vi "time + theta.vi"(5 "Draw Area Size":cluster{"Width":u32, "Height":u32}={"Width"=800, "Height"=90}, 6 "Sample volumes":dbl[unit][](array[numeric]) format="%.2f", 7 "colors":u32[](array[colorbox])=[16717824, 16775680, 65289, 1442031, 16711898, 9306367, 16711704, 16773418, 4914944, 65469, 18175, 15805183, 16711776, 16745216, 16773632, 7396352, 62719, 16383, 15925503, 16711686, 16775954, 65372, 51354, 19711, 7082751, 15663288, 16711680, 11468586, 52719, 1214975, 16711830], 8 "Sample start times":dbl[unit][](array[numeric]) format="%<%H:%M:%S>t", 9 "State Settings":T2[][](array[typedef]) {"valve cycle time" min=0.2 step=0.1 format="%.2f"; "flow division"."5" min=0.0 max=1.0 step=0.01 format="%.3f"; "flow division"."4" min=0.0 max=1.0 step=0.01 format="%.3f"; "flow division"."3" min=0.0 max=1.0 step=0.01 format="%.3f"; "flow division"."2" min=0.0 max=1.0 step=0.01 format="%.3f"; "flow division"."1" min=0.0 max=1.0 step=0.01 format="%.3f"; "flow rate" format="%.3f"}, 10 "Cycle list":i32(listbox), 11 "Method settings":T5 {"Column"."porosity" format="%.4f"; "Column"."diameter" format="%.2f"; "Column"."length" format="%.2f"}) -> (0 "Samples":T1, 2 "Sample plot":picture, 3 "tout":dbl[unit][](array[numeric]))   [LabVIEW 2012]
uses:
  Method settings.ctl
  Peristaltic/3-stop colors.ctl
  State Setting.ctl
  Stamp/Switch settings vertical.ctl
  flow fraction.ctl
  Samples.ctl
panel:
  out "f":dbl[](array[numeric])
  out "tcum":dbl[unit][](array[numeric])
  out "theta":dbl[unit][](array[numeric])
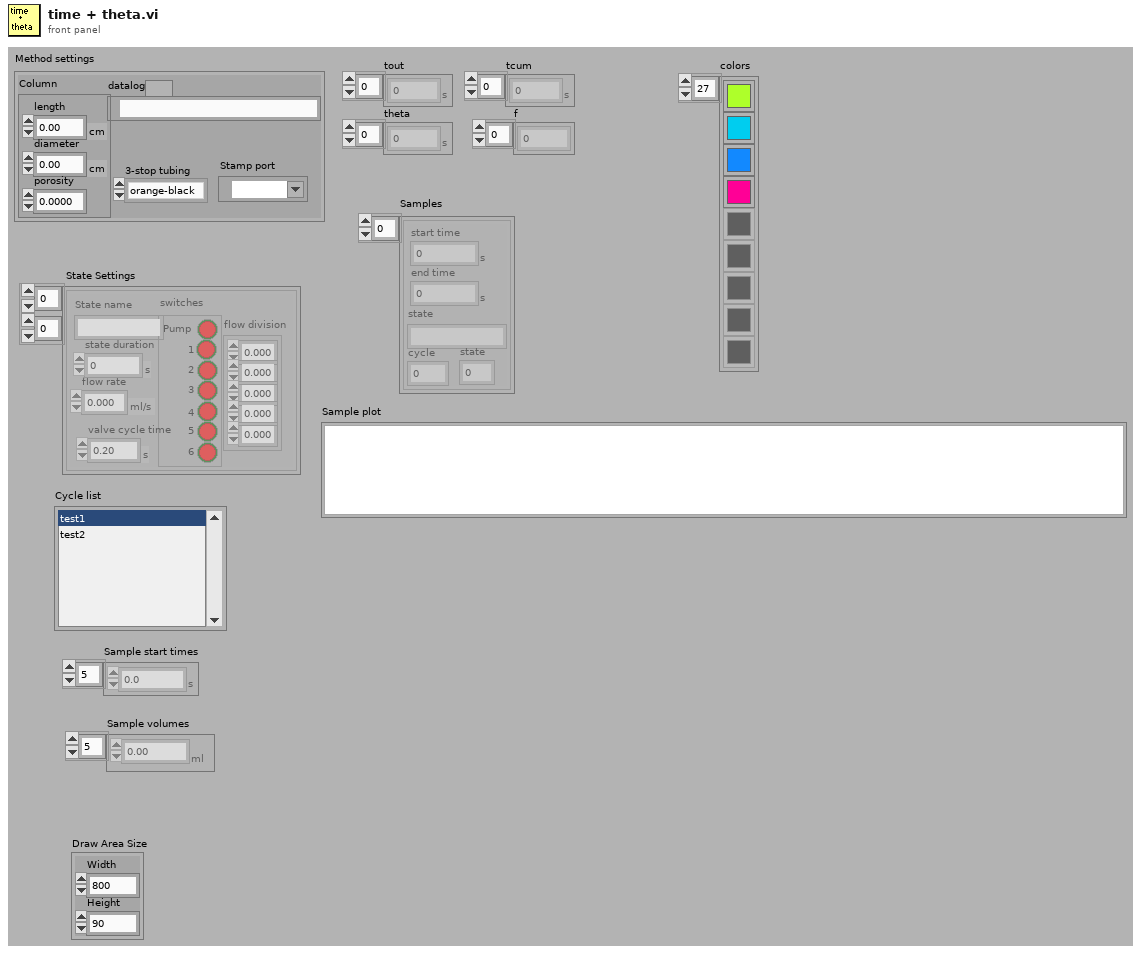
[diagram p1: front panel]
types:
  T1 = typedef "Samples.ctl" = cluster{"start time":dbl[unit], "end time":dbl[unit], "state":string, "cycle":u16, "state":u16}[]
  T2 = typedef "State Setting.ctl" = cluster{"switches":T3, "flow rate":dbl[unit], "flow division":cluster{"1":T4, "2":T4, "3":T4, "4":T4, "5":T4}, "State name":string, "state duration":dbl[unit], "valve cycle time":dbl[unit]}
  T3 = typedef "Switch settings vertical.ctl" = cluster{"Pump":bool, "1":bool, "2":bool, "3":bool, "4":bool, "5":bool, "6":bool}
  T4 = typedef "flow fraction.ctl" = dbl
  T5 = typedef "Method settings.ctl" = cluster{"3-stop tubing":T6, "Stamp port":refnum<visa-resource-name>, "datalog":path, "Column":cluster{"length":dbl[unit], "diameter":dbl[unit], "porosity":dbl}}
  T6 = typedef "3-stop colors.ctl" = enum16{"orange-black", "orange-red", "orange-blue", "orange-green", "green-yellow", "orange-yellow", "white-yellow", "orange-white", "black-black", "orange-orange", "white-black", "white-white", "white-red", "red-red", "red-grey", "grey-grey", "yellow-yellow", "yellow-blue", "blue-blue", "blue-green", "green-green", "purple-purple", "purple-black", "purple-orange", "purple-white", "black-white", "13", "14", "15", "16", "17", "18"}
  T7 = cluster{"Numeric":dbl[unit], dbl[unit], "State name":string, dbl, dbl}
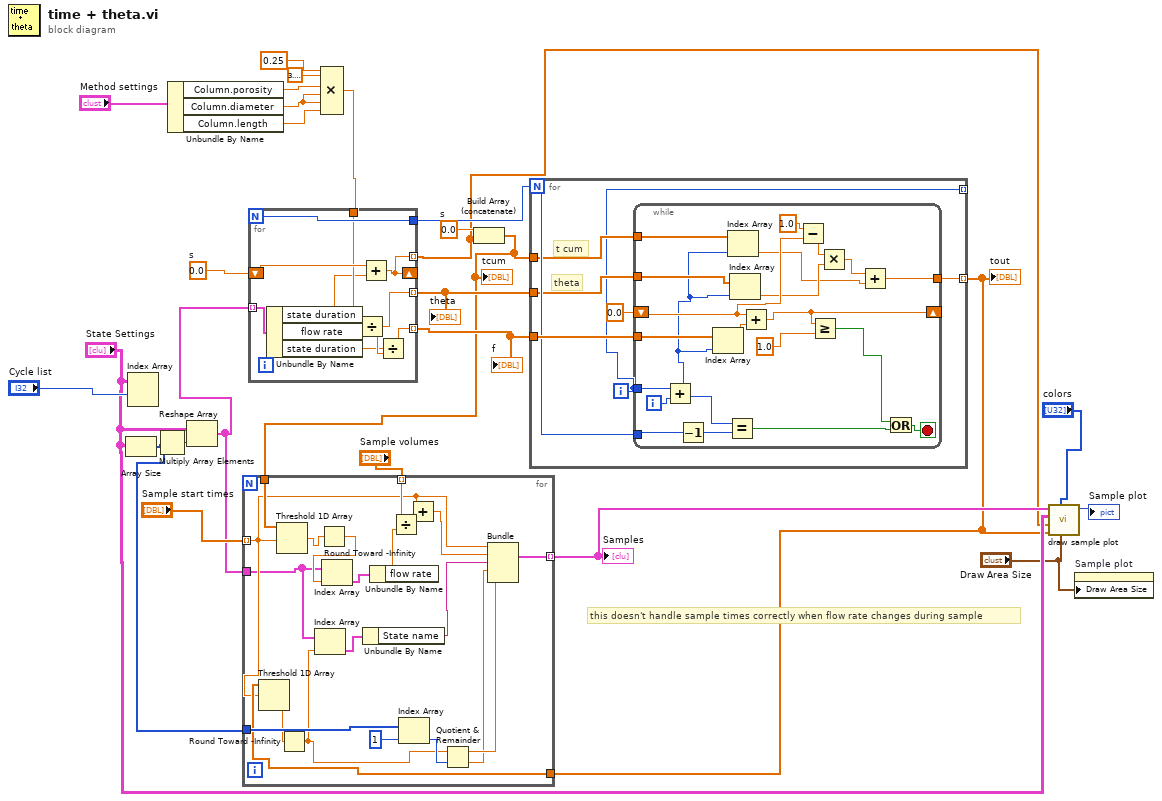
[diagram p0: block diagram]
diagram:
  w15 = dbl[unit] 0.0  # s
  w17 = dbl[unit] 0.0  # s
  # "this doesn't handle sample times correctly when flow rate changes during sample"
  n1 = Array Size(array="State Settings") -> (size(s)=w9:i32[])
  n2 = Index Array(array="State Settings", index (row)="Cycle list") -> ()  [unwired: 1 in, 1 out]
  n3 = Multiply Array Elements(1:w9) -> (0:w11:i32)
  n4 = Unbundle By Name("Method settings") -> ("Column.porosity"=w23:dbl, "Column.diameter"=w24:dbl[unit], "Column.length"=w25:dbl[unit])
  n5 = Reshape Array("State Settings", w11) -> (w10:T2[])
  n6 = Compound Arithmetic op=MULTIPLY(0.25 ("value"), 3.141592653589793, w23, w24, w24, w25) -> (w19:dbl[unit])
  n7 = for {
    N -> [w35]
    tunnel: w10 -> [w36] mode=indexing
    tunnel: w19 -> [w33]
    tunnel: [w32] -> w14 mode=indexing
    tunnel: [w35] -> w18
    shift-right: [w27] -> _
    shift-left: w17 -> [w34]
    tunnel: [w27] -> w4 mode=indexing
    tunnel: [w30] -> w16 mode=indexing
    n8 = Unbundle By Name(w36) -> ("state duration"=w31:dbl[unit], "flow rate"=w28:dbl[unit], "state duration"=w29:dbl[unit])
    n9 = Divide(x=w33, y=w28) -> (x/y=w30:dbl[unit])
    n10 = Add(x=w34, y=w31) -> (x+y=w27:dbl[unit])
    n11 = Divide(x=w29, y=w30) -> (x/y=w32:dbl)
  }
  "theta" <- w16
  "f" <- w14
  n12 = Build Array (concatenate)(w15, w4) -> (w3:dbl[unit][])
  "tcum" <- w3
  n13 = for {
    N: w18 -> [w42]
    tunnel: w14 -> [w43]
    tunnel: w3 -> [w40]
    tunnel: w16 -> [w39]
    tunnel: [w38] -> w2 mode=indexing
    tunnel: [w37] -> _ mode=indexing
    i -> [w37]
    # "t cum"
    # "theta"
    n14 = while {
      tunnel: w43 -> [w64]
      tunnel: w37 -> [w62]
      tunnel: w42 -> [w60]
      shift-right: [w46] -> _
      shift-left: 0.0 -> [w52]
      tunnel: w40 -> [w57]
      tunnel: w39 -> [w56]
      tunnel: [w55] -> w38
      i -> [w63]
      stop <- w61 stop-if-true
      n15 = Add(x=w62, y=w63) -> (x+y=w51:i32)
      n16 = Decrement(x=w60) -> (x-1=w54:i32)
      n17 = Index Array(array=w64, index=w51) -> (element=w58:dbl)
      n18 = Equal?(x=w51, y=w54) -> (x = y?=w59:bool)
      n19 = Index Array(array=w57, index=w51) -> (element=w47:dbl[unit])
      n20 = Index Array(array=w56, index=w51) -> (element=w49:dbl[unit])
      n21 = Add(x=w52, y=w58) -> (x+y=w46:dbl)
      n22 = Subtract(x=1.0 ("y"), y=w52) -> (x-y=w50:dbl)
      n23 = Greater Or Equal?(x=w46, y=1.0) -> (x >= y?=w44:bool)
      n24 = Multiply(x=w50, y=w49) -> (x*y=w48:dbl[unit])
      n25 = Add(x=w48, y=w47) -> (x+y=w55:dbl[unit])
      n26 = Or(x=w44, y=w59) -> (x .or. y?=w61:bool)
    }
  }
  "tout" <- w2
  n27 = for {
    tunnel: w3 -> [w85]
    tunnel: "Sample start times" -> [w69] mode=indexing
    tunnel: "Sample volumes" -> [w84] mode=indexing
    tunnel: w10 -> [w67]
    tunnel: [w82] -> w8 mode=indexing
    tunnel: w9 -> [w77]
    tunnel: w2 -> [w72]
    n28 = Threshold 1D Array(2:w69, 3:w72) -> (0:w73:dbl)  [unwired: 1 in]
    n29 = Threshold 1D Array(2:w69, 3:w85) -> (0:w75:dbl)  [unwired: 1 in]
    n30 = Round Toward -Infinity(1:w73) -> (0:w68:dbl)
    n31 = Index Array(array=w67, index=w68) -> (element=w66:T2)
    n32 = Round Toward -Infinity(1:w75) -> (0:w71:dbl)
    n33 = Index Array(array=w67, index=w71) -> (element=w83:T2)
    n34 = Unbundle By Name(w66) -> ("State name"=w65:string)
    n35 = Unbundle By Name(w83) -> ("flow rate"=w81:dbl[unit])
    n36 = Divide(x=w84, y=w81) -> (x/y=w80:dbl[unit])
    n37 = Index Array(array=w77, index=1) -> (element=w74:i32)
    n38 = Add(x=w69, y=w80) -> (x+y=w79:dbl[unit])
    n39 = Quotient & Remainder(x=w68, y=w74) -> (x-y*floor(x/y)=w76:dbl, floor(x/y)=w70:dbl)
    n40 = Bundle("Numeric"=w69, w79, "State name"=w65, w70, w76) -> (w82:T7)  [unwired: 1 in]
  }
  "Samples" <- w8
  n41 = call "draw sample plot.vi"("Draw Area Size"="Draw Area Size", "colors"="colors", "tout"=w2, "tcum"=w4, "State Settings"="State Settings", "Samples"=w8) -> ("Sample plot"=→"Sample plot":picture)  [unwired: 5 in]
  n42 = property on="Sample plot" class="Pict"("Draw Area Size"="Draw Area Size") -> ()  [unwired: 2 in, 2 out]
